vi "Read Magnetic Deviation Msg.vi"(8 "error in (no error)":errorcluster, 11 "Set Mag Dev Message in":refnum<class "Set Mag Dev Message.lvclass">) -> (0 "error out":errorcluster, 2 "Magnetic Deviation":dbl, 3 "Set Mag Dev Message out":refnum<class "Set Mag Dev Message.lvclass">)   [LabVIEW 2015, in "RDS Child Messages.lvlib" / "Set Mag Dev Message.lvclass"]
uses:
  Set Mag Dev Message.lvclass
  Set Mag Dev Message.lvclass/Set Mag Dev Message.ctl
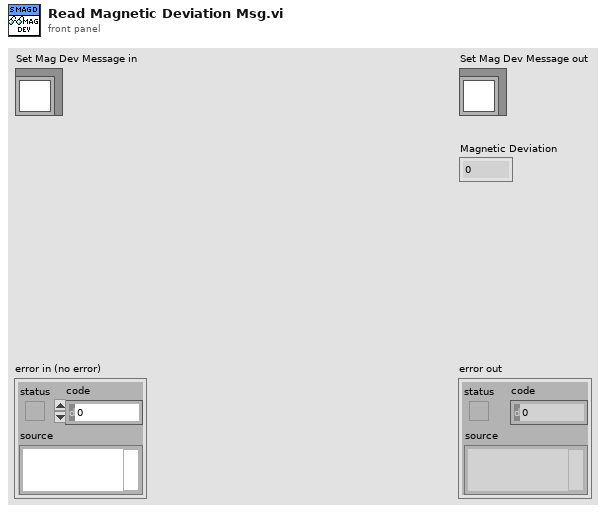
[diagram p1: front panel]
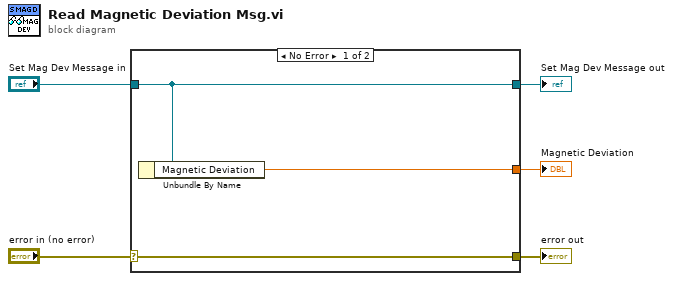
[diagram p0: block diagram]
diagram:
  n1 = case shown="No Error" "error in (no error)" {
    selector: "error in (no error)" -> [w8 w9]
    tunnel: [w8 w9] -> w4
    tunnel: [w7 w10] -> w2
    tunnel: "Set Mag Dev Message in" -> [w7 w10]
    tunnel: [w6 _] -> w1
    frame No Error {
      n2 = Unbundle By Name(w7) -> ("Magnetic Deviation"=w6:dbl)
    }
    frame Error {
    }
  }
  "error out" <- w4
  "Set Mag Dev Message out" <- w2
  "Magnetic Deviation" <- w1
